vi "Write Calibration config to file.vi"(8 "error in (no error)":errorcluster, 10 "configuration file path":path, 11 "Calibration config.":T1) -> (0 "error out":errorcluster)   [LabVIEW 2017]
uses:
  Typedefs/Calibration config.ctl
  Typedefs/Objective Config.ctl
  Typedefs/Prechirper Cal Config.ctl
  Typedefs/PreChirper constants.ctl
  <vilib>/Utility/config.llb/Write Key (String).vi
  <vilib>/Utility/config.llb/Write Key (Double).vi
  <vilib>/Utility/config.llb/Write Key (Boolean).vi
  <vilib>/Utility/config.llb/Write Key (I32).vi
  <vilib>/Utility/config.llb/NI_LVConfig.lvlib
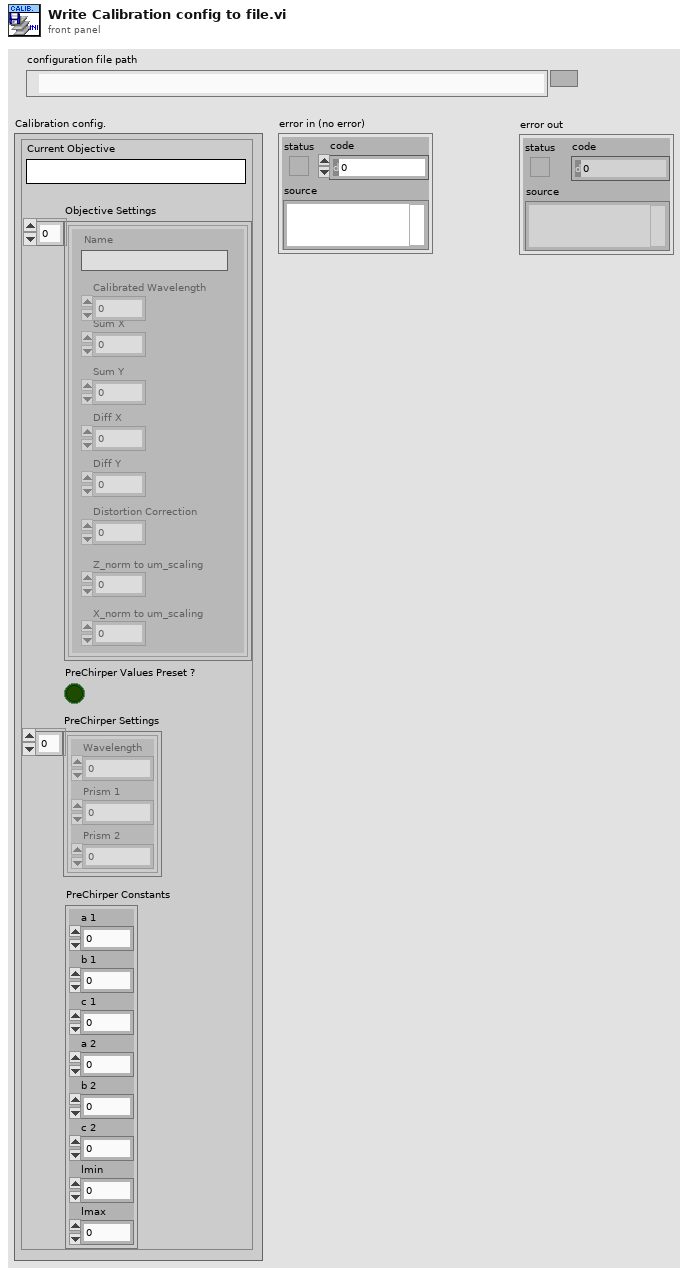
[diagram p1: front panel]
types:
  T1 = typedef "Calibration config.ctl" = cluster{"Current Objective":string, "Objective Settings":T2[], "PreChirper Values Preset ?":bool, "PreChirper Settings":T3[], "PreChirper Constants":T4}
  T2 = typedef "Objective Config.ctl" = cluster{"Name":string, "Sum X":dbl, "Sum Y":dbl, "Diff X":dbl, "Diff Y":dbl, "Distortion Correction":dbl, "Z_norm to um_scaling":dbl, "X_norm to um_scaling":dbl, "Calibrated Wavelength":dbl}
  T3 = typedef "Prechirper Cal Config.ctl" = cluster{"Wavelength":i32, "Prism 1":i32, "Prism 2":i32}
  T4 = typedef "PreChirper constants.ctl" = cluster{"a 1":i32, "b 1":i32, "c 1":i32, "a 2":i32, "b 2":i32, "c 2":i32, "lmin":i32, "lmax":i32}
  T5 = typedef "NI_LVConfig.lvlib/Config Data RefNum.ctl" = refnum<k1>
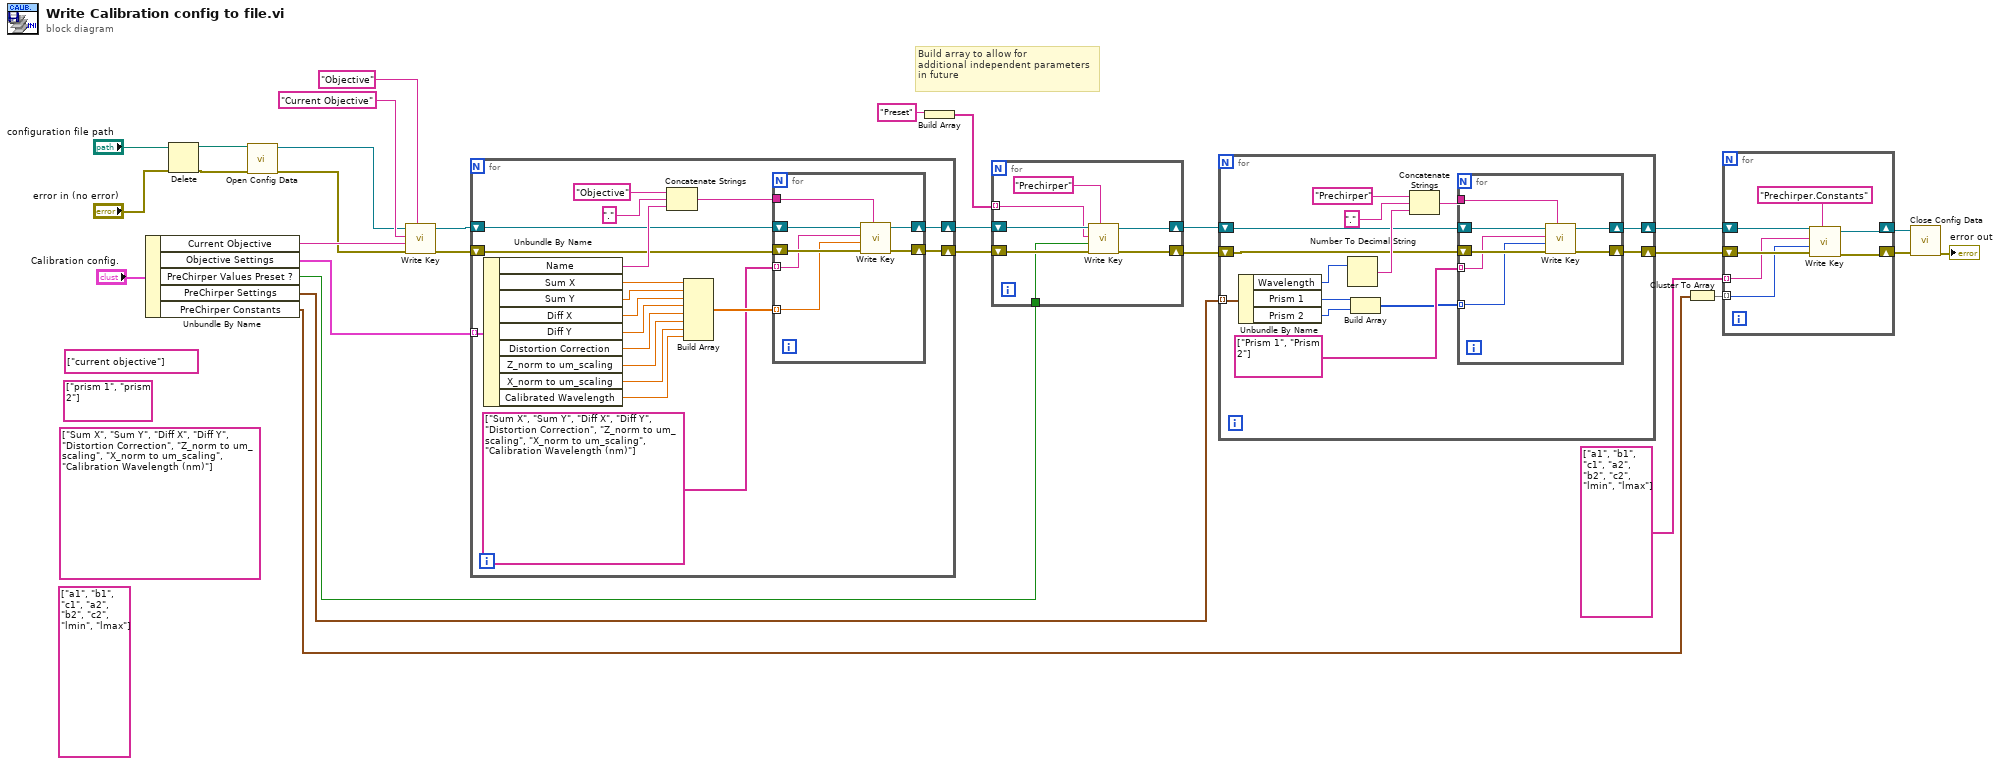
[diagram p0: block diagram]
diagram:
  (unwired) string[] ["a1", "b1", "c1", "a2", "b2", "c2", "lmin", "lmax"]
  (unwired) string[] ["Sum X", "Sum Y", "Diff X", "Diff Y", "Distortion Correction", "Z_norm to um_scaling", "X_norm to um_scaling", "Calibration Wavelength (nm)"] ("array (last n elements first)")
  (unwired) string[] ["prism 1", "prism 2"]
  (unwired) string[] ["current objective"]
  # "Build array to allow for \nadditional independent parameters\nin future"
  n1 = Unbundle By Name("Calibration config.") -> ("Current Objective"=w27:string, "Objective Settings"=w22:T2[], "PreChirper Values Preset ?"=w12:bool, "PreChirper Settings"=w13:T3[], "PreChirper Constants"=w7:T4)
  n2 = Delete(path (use dialog)="configuration file path", error in="error in (no error)") -> (deleted path=w16:path, error out=w18:errorcluster)  [unwired: 3 in, 1 out]
  n3 = call <vilib>:"Open Config Data.vi"("error in (no error)"=w18, "configuration file path"=w16) -> ("error out"=w24:errorcluster, "refnum"=w25:T5)  [unwired: 7 in, 1 out]
  n4 = call-poly <vilib>:"Write Key.vi"("section"="Objective", "error in (no error)"=w24, "value"=w27, "key"="Current Objective", "refnum"=w25) -> ("error out"=w21:errorcluster, "refnum out"=w23:T5)  [unwired: 4 in, 1 out]
  n5 = for {
    tunnel: w22 -> [w48] mode=indexing
    shift-right: [w32] -> w14
    shift-left: w23 -> [w34]
    shift-right: [w30] -> w15
    shift-left: w21 -> [w31]
    n6 = Unbundle By Name(w48) -> ("Name"=w45:string, "Sum X"=w44:dbl, "Sum Y"=w43:dbl, "Diff X"=w42:dbl, "Diff Y"=w41:dbl, "Distortion Correction"=w40:dbl, "Z_norm to um_scaling"=w39:dbl, "X_norm to um_scaling"=w38:dbl, "Calibrated Wavelength"=w37:dbl)
    n7 = Concatenate Strings("Objective" ("section"), "." ("string"), w45) -> (w33:string)
    n8 = Build Array(w44, w43, w42, w41, w40, w39, w38, w37) -> (w36:dbl[])
    n9 = for {
      tunnel: w36 -> [w52] mode=indexing
      tunnel: string[] ["Sum X", "Sum Y", "Diff X", "Diff Y", "Distortion Correction", "Z_norm to um_scaling", "X_norm to um_scaling", "Calibration Wavelength (nm)"] ("array (last n elements first)") -> [w53] mode=indexing
      tunnel: w33 -> [w51]
      shift-right: [w50] -> w32
      shift-left: w34 -> [w55]
      shift-right: [w49] -> w30
      shift-left: w31 -> [w54]
      n10 = call-poly <vilib>:"Write Key.vi"("section"=w51, "error in (no error)"=w54, "value"=w52, "key"=w53, "refnum"=w55) -> ("error out"=w49:errorcluster, "refnum out"=w50:T5)  [unwired: 4 in, 1 out]
    }
  }
  n11 = Build Array("Preset" ("key")) -> (w1:string[])
  n12 = for {
    shift-right: [w61] -> w11
    shift-left: w15 -> [w62]
    shift-right: [w59] -> w10
    shift-left: w14 -> [w60]
    tunnel: w12 -> [w57]
    tunnel: w1 -> [w56] mode=indexing
    n13 = call-poly <vilib>:"Write Key.vi"("section"="Prechirper", "error in (no error)"=w62, "value"=w57, "key"=w56, "refnum"=w60) -> ("error out"=w61:errorcluster, "refnum out"=w59:T5)  [unwired: 4 in, 1 out]
  }
  n14 = for {
    tunnel: w13 -> [w74] mode=indexing
    shift-right: [w68] -> w9
    shift-left: w11 -> [w70]
    shift-right: [w69] -> w8
    shift-left: w10 -> [w71]
    n15 = Unbundle By Name(w74) -> ("Wavelength"=w73:i32, "Prism 1"=w65:i32, "Prism 2"=w64:i32)
    n16 = Number To Decimal String(number=w73) -> (decimal integer string=w72:string)  [unwired: 1 in]
    n17 = Build Array(w65, w64) -> (w63:i32[])
    n18 = Concatenate Strings("Prechirper" ("section"), "." ("string"), w72) -> (w67:string)
    n19 = for {
      tunnel: w63 -> [w80] mode=indexing
      tunnel: string[] ["Prism 1", "Prism 2"] -> [w81] mode=indexing
      tunnel: w67 -> [w79]
      shift-right: [w78] -> w69
      shift-left: w71 -> [w83]
      shift-right: [w77] -> w68
      shift-left: w70 -> [w82]
      n20 = call-poly <vilib>:"Write Key.vi"("section"=w79, "error in (no error)"=w82, "value"=w80, "key"=w81, "refnum"=w83) -> ("error out"=w77:errorcluster, "refnum out"=w78:T5)  [unwired: 4 in, 1 out]
    }
  }
  n21 = Cluster To Array(cluster=w7) -> (array=w5:i32[])
  n22 = for {
    shift-right: [w85] -> w4
    shift-left: w9 -> [w90]
    shift-right: [w84] -> w3
    shift-left: w8 -> [w89]
    tunnel: string[] ["a1", "b1", "c1", "a2", "b2", "c2", "lmin", "lmax"] -> [w86] mode=indexing
    tunnel: w5 -> [w87] mode=indexing
    n23 = call-poly <vilib>:"Write Key.vi"("section"="Prechirper.Constants", "error in (no error)"=w90, "value"=w87, "key"=w86, "refnum"=w89) -> ("error out"=w85:errorcluster, "refnum out"=w84:T5)  [unwired: 4 in, 1 out]
  }
  n24 = call <vilib>:"Close Config Data.vi"("error in (no error)"=w4, "refnum"=w3) -> ("error out"=→"error out":errorcluster)  [unwired: 8 in, 1 out]
